vi "Write Measured Phase.vi"(8 "error in (no error)":errorcluster, 10 "Abs_Double Float.lvclass":refnum<class "Abs_Double Float.lvclass">, 11 "Measure Waveform in":refnum<class "Measure Waveform.lvclass">) -> (0 "error out":errorcluster, 3 "Measure Waveform out":refnum<class "Measure Waveform.lvclass">)   [LabVIEW 2021, in "Measure Waveform.lvclass"]
uses:
  Measure Waveform.lvclass
  <vilib>/TSA/Abstract Data Classes/Abs_Types/Double Float/Abs_Double Float.lvclass
  Measure Waveform.lvclass/Measure Waveform.ctl
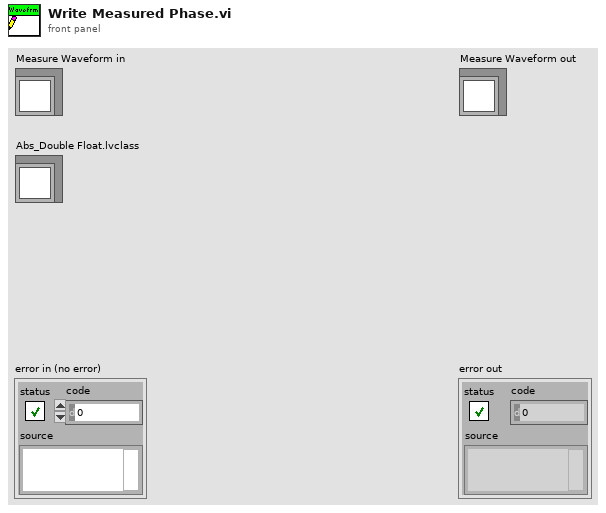
[diagram p1: front panel]
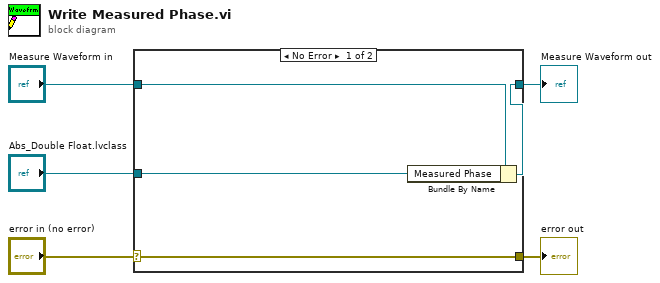
[diagram p0: block diagram]
diagram:
  n1 = case shown="No Error" "error in (no error)" {
    selector: "error in (no error)" -> [w9 w10]
    tunnel: [w9 w10] -> w4
    tunnel: [w7 w11] -> w2
    tunnel: "Measure Waveform in" -> [w8 w11]
    tunnel: "Abs_Double Float.lvclass" -> [w6 _]
    frame No Error {
      n2 = Bundle By Name(cluster=w8, "Measured Phase"=w6) -> (w7:refnum<class "Measure Waveform.lvclass">)
    }
    frame Error {
    }
  }
  "error out" <- w4
  "Measure Waveform out" <- w2
